vi "Kettle.vi"(10 "M":fxp<+,32,32>=3400000.0, 11 "Trigger":bool) -> (3 "Kettle 1 Out":fxp<+/-,8,8>)   [LabVIEW 2015]
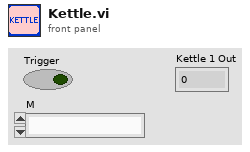
[diagram p1: front panel]
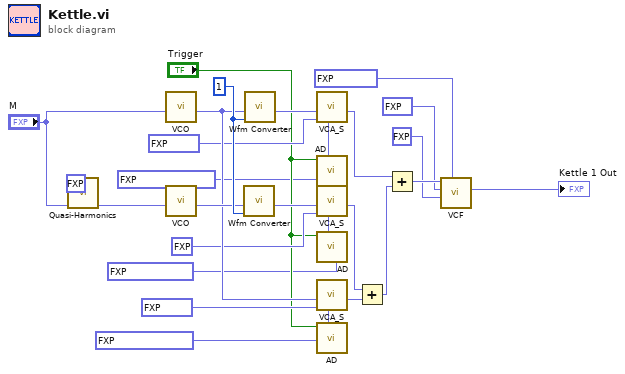
[diagram p0: block diagram]
diagram:
  w23 = u8 1 ("select")
  n1 = call "Quasi-Harmonics.vi"("Relative Freq"=fxp<+,8,3> 2.0 ("relative f 2"), "1st partial"="M") -> ("Result Partial"=w26:fxp<+,32,32>)  [unwired: 9 in]
  n2 = call "VCO.vi"("M"="M") -> ("Sine Sample"=w11:fxp<+/-,8,8>)  [unwired: 10 in]
  n3 = call "VCO.vi"("M"=w26) -> ("Sine Sample"=w12:fxp<+/-,8,8>)  [unwired: 10 in]
  n4 = call "Wfm Converter.vi"("Select"=w23, "Sample In"=w12) -> ("Sample Out"=w22:fxp<+/-,8,8>)  [unwired: 9 in]
  n5 = call "Wfm Converter.vi"("Select"=w23, "Sample In"=w11) -> ("Sample Out"=w24:fxp<+/-,8,8>)  [unwired: 9 in]
  n6 = call "AD.vi"("1/Decay"=fxp<+,16,0> 1.52587890625e-05, "Trigger"="Trigger") -> ("Sample Out"=w6:fxp<+,8,0>)  [unwired: 9 in]
  n7 = call "VCA_S.vi"("EG"=w6, "Amount"=fxp<+,8,0> 0.99609375, "Sample In"=w24) -> ("Sample Out"=w25:fxp<+/-,8,8>)  [unwired: 8 in]
  n8 = call "AD.vi"("1/Decay"=fxp<+,16,0> 6.103515625e-05 ("1/Decay 3"), "Trigger"="Trigger") -> ("Sample Out"=w4:fxp<+,8,0>)  [unwired: 9 in]
  n9 = call "VCA_S.vi"("EG"=w4, "Amount"=fxp<+,8,0> 0.5, "Sample In"=w22) -> ("Sample Out"=w16:fxp<+/-,8,8>)  [unwired: 8 in]
  n10 = call "AD.vi"("1/Decay"=fxp<+,16,0> 1.52587890625e-05 ("1/Decay 3"), "Trigger"="Trigger") -> ("Sample Out"=w2:fxp<+,8,0>)  [unwired: 9 in]
  n11 = call "VCA_S.vi"("EG"=w2, "Amount"=fxp<+,8,0> 0.8984375, "Sample In"=w11) -> ("Sample Out"=w15:fxp<+/-,8,8>)  [unwired: 8 in]
  n12 = Add(x=w16, y=w15) -> (x+y=w14:fxp<+/-,8,8>)
  n13 = Add(x=w25, y=w14) -> (x+y=w21:fxp<+/-,8,8>)
  n14 = call "VCF.vi"("Amount"=fxp<+,8,0> 0.99609375, "Q1"=fxp<+/-,18,18> 1.0, "F1"=fxp<+/-,18,18> 1500.0, "Sample In"=w21) -> ("LP Out"=→"Kettle 1 Out":fxp<+/-,8,8>)  [unwired: 5 in, 2 out]
